vi "PatchForRelease.vi"   [LabVIEW 2013, in "Advanced Plotting Toolkit.lvlib"]
uses:
  Advanced Plotting Toolkit.lvlib
  priv/Python.vi
  Config.vi
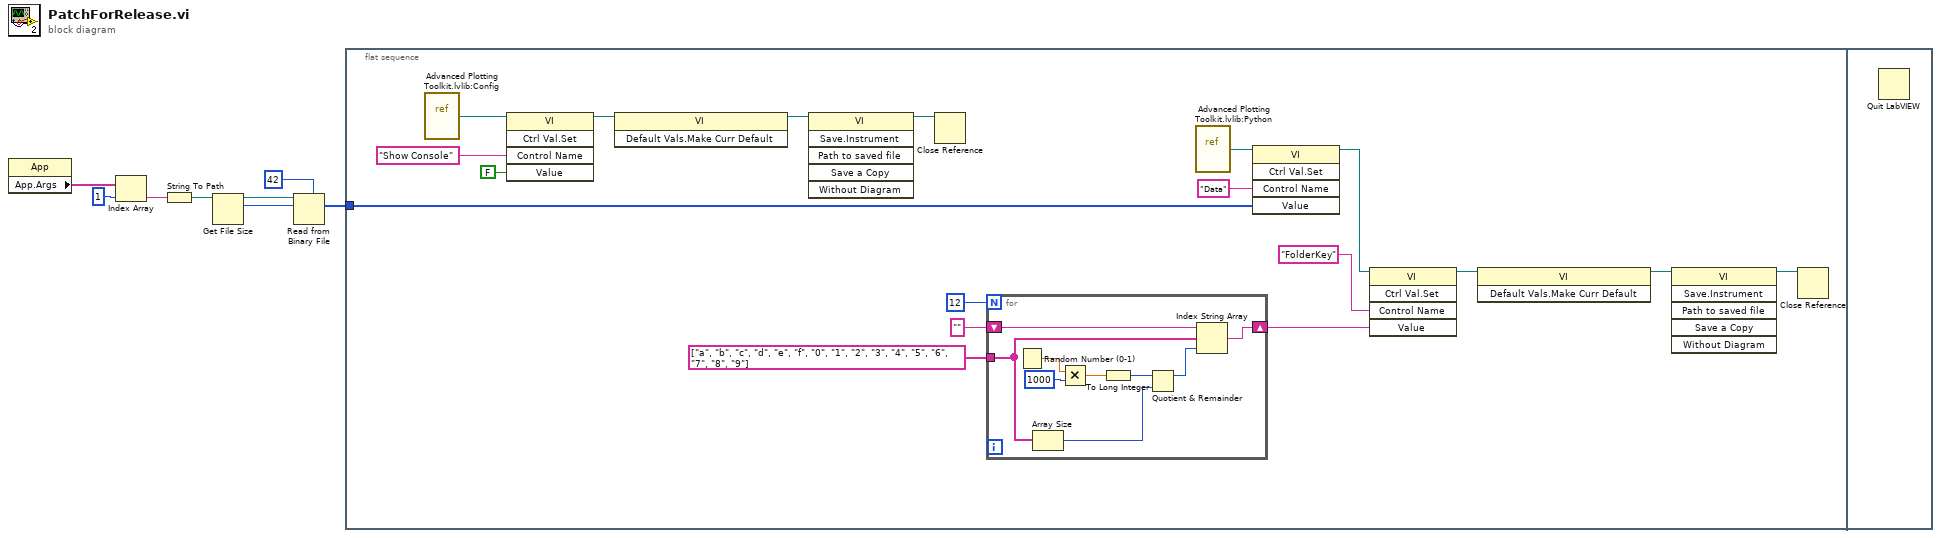
[diagram p0: block diagram]
diagram:
  n1 = property class="App"() -> ("App.Args"=w8:string[])  [unwired: 2 in, 2 out]
  n2 = Index Array(array=w8, index=1) -> (element=w6:string)
  n3 = String To Path(string=w6) -> (path=w4:path)
  n4 = Get File Size(file=w4) -> (refnum out=w3:refnum<file>, size (in bytes)=w1:i64)  [unwired: 1 in, 1 out]
  n5 = Read from Binary File(5:u8 42, 10:w1, 11:w3) -> (2:w5:u8[])  [unwired: 3 in, 3 out]
  n6 = flat-sequence {
    tunnel: w5 -> [w22]
    frame #0 {
      n7 = vi-ref "Advanced Plotting Toolkit.lvlib:Config.vi"() -> (w17:refnum<vi>)
      n8 = invoke class="VI" method="Ctrl Val.Set"(reference=w17, "Control Name"="Show Console", "Value"=FALSE) -> (reference out=w20:refnum<vi>)  [unwired: 2 in, 4 out]
      n9 = invoke class="VI" method="Default Vals.Make Curr Default"(reference=w20) -> (reference out=w19:refnum<vi>)  [unwired: 2 in, 2 out]
      n10 = invoke class="VI" method="Save.Instrument"(reference=w19) -> (reference out=w18:refnum<vi>)  [unwired: 5 in, 5 out]
      n11 = Close Reference(reference=w18) -> ()  [unwired: 1 in, 1 out]
      n12 = for {
        N: 12 -> [_]
        tunnel: string[] ["a", "b", "c", "d", "e", "f", "0", "1", "2", "3", "4", "5", "6", "7", "8", "9"] -> [w31]
        shift-right: [w34] -> w9
        shift-left: "" ("String") -> [w35]
        n13 = Random Number (0-1)() -> (number: 0 to 1=w33:dbl)
        n14 = Array Size(array=w31) -> (size(s)=w30:i32)
        n15 = Multiply(x=w33, y=1000) -> (x*y=w29:dbl)
        n16 = To Long Integer(number=w29) -> (32bit integer=w28:i32)
        n17 = Quotient & Remainder(x=w28, y=w30) -> (x-y*floor(x/y)=w27:i32)  [unwired: 1 out]
        n18 = Index String Array(1:w27, 2:w31, 3:w35) -> (0:w34:string)
      }
      n19 = vi-ref "Advanced Plotting Toolkit.lvlib:Python.vi"() -> (w23:refnum<vi>)
      n20 = invoke class="VI" method="Ctrl Val.Set"(reference=w23, "Control Name"="Data", "Value"=w22) -> (reference out=w15:refnum<vi>)  [unwired: 2 in, 4 out]
      n21 = invoke class="VI" method="Ctrl Val.Set"(reference=w15, "Control Name"="FolderKey", "Value"=w9) -> (reference out=w14:refnum<vi>)  [unwired: 2 in, 4 out]
      n22 = invoke class="VI" method="Default Vals.Make Curr Default"(reference=w14) -> (reference out=w25:refnum<vi>)  [unwired: 2 in, 2 out]
      n23 = invoke class="VI" method="Save.Instrument"(reference=w25) -> (reference out=w24:refnum<vi>)  [unwired: 5 in, 5 out]
      n24 = Close Reference(reference=w24) -> ()  [unwired: 1 in, 1 out]
    }
    frame #1 {
      n25 = Quit LabVIEW() -> ()  [unwired: 1 in]
    }
  }
